vi "Errors.vi"() -> ()   [LabVIEW 2022 SP3]
uses:
  <vilib>/Utility/error.llb/DialogType.ctl
panel:
  out "source":string
  out "code":i32
  out "status":bool
  out "String":string
  in  "Path":path
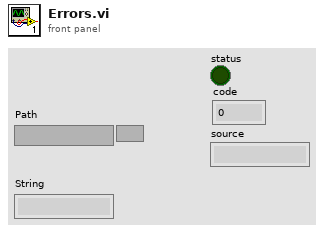
[diagram p1: front panel]
types:
  T1 = typedef "DialogType.ctl" = u16
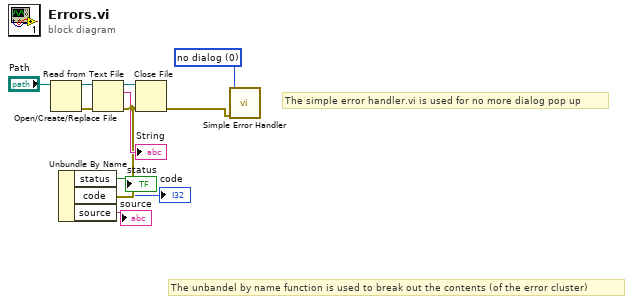
[diagram p0: block diagram]
diagram:
  w1 = T1 0 items=["no dialog", "OK message", "continue or stop message", "OK message + warnings", "continue/stop + warnings"] ("type of dialog (OK msg:1)")
  # "The simple error handler.vi is used for no more dialog pop up"
  # "The unbandel by name function is used to break out the contents (of the error cluster)"
  n1 = Open/Create/Replace File(file path (use dialog)="Path") -> (refnum out=w10:refnum<file>, error out=w7:errorcluster)  [unwired: 5 in, 1 out]
  n2 = Read from Text File(file (use dialog)=w10, error in=w7) -> (refnum out=w9:refnum<file>, text=→"String":string, error out=w6:errorcluster)  [unwired: 2 in, 1 out]
  n3 = Unbundle By Name(w6) -> ("status"=→"status":bool, "code"=→"code":i32, "source"=→"source":string)
  n4 = Close File(refnum=w9, error in=w6) -> (error out=w2:errorcluster)  [unwired: 1 out]
  n5 = call <vilib>:"Simple Error Handler.vi"("type of dialog (OK msg:1)"=w1, "error in (no error)"=w2) -> ()  [unwired: 3 in, 5 out]
